vi "ENPH354_LabSCPE_dVdI-(SubVI).vi"(9 "Shunt or Series":bool, 10 "Current in":dbl[](array[numeric]), 11 "Voltage in":dbl[](array[numeric])) -> (2 "dV/dI":dbl, 3 "IDX":u8)   [LabVIEW 2020]
panel:
  # "TRUE: Shunt Resistance\nFALSE: Series Resistance"
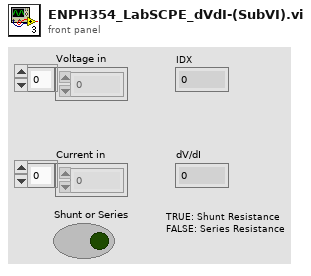
[diagram p1: front panel]
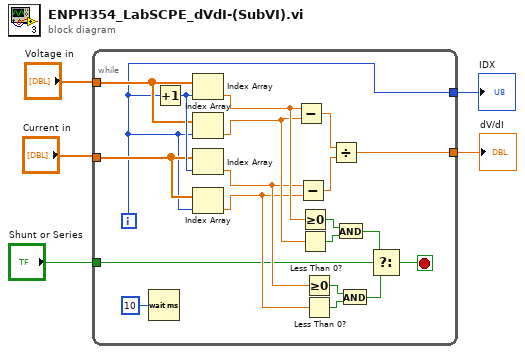
[diagram p0: block diagram]
diagram:
  n1 = while {
    tunnel: "Voltage in" -> [w22]
    tunnel: "Current in" -> [w21]
    tunnel: "Shunt or Series" -> [w9]
    tunnel: [w8] -> w4
    tunnel: [w7] -> w5
    i -> [w7]
    stop <- w10 stop-if-true
    n2 = Wait (ms)(milliseconds to wait=u32 10) -> ()  [unwired: 1 out]
    n3 = Increment(x=w7) -> (x+1=w23:i32)
    n4 = Index Array(array=w22, index=w23) -> (element=w15:dbl)
    n5 = Index Array(array=w22, index=w7) -> (element=w14:dbl)
    n6 = Index Array(array=w21, index=w23) -> (element=w12:dbl)
    n7 = Index Array(array=w21, index=w7) -> (element=w11:dbl)
    n8 = Subtract(x=w15, y=w14) -> (x-y=w25:dbl)
    n9 = Subtract(x=w12, y=w11) -> (x-y=w24:dbl)
    n10 = Greater Or Equal To 0?(x=w15) -> (x >= 0?=w20:bool)
    n11 = Less Than 0?(x=w14) -> (x < 0?=w19:bool)
    n12 = Greater Or Equal To 0?(x=w12) -> (x >= 0?=w17:bool)
    n13 = Less Than 0?(x=w11) -> (x < 0?=w16:bool)
    n14 = Divide(x=w25, y=w24) -> (x/y=w8:dbl)
    n15 = And(x=w20, y=w19) -> (x .and. y?=w18:bool)
    n16 = And(x=w17, y=w16) -> (x .and. y?=w13:bool)
    n17 = Select(t=w18, s=w9, f=w13) -> (s? t:f=w10:bool)
  }
  "IDX" <- w5
  "dV/dI" <- w4
